vi "通过引用调用VI.vi"() -> ()   [LabVIEW 2013]
uses:
  <vilib>/Platform/TimedLoop/XDataNode/timing_clust.ctl
  <vilib>/Platform/TimedLoop/XDataNode/nitl_modes.ctl
  <vilib>/Platform/TimedLoop/XDataNode/wakeup.ctl
  <vilib>/Platform/TimedLoop/XDataNode/XDataNode.xnode
  <vilib>/Platform/TimedLoop/XDataNode/XDNodeRunTimeDep.lvlib
panel:
  in  "关闭引用":bool
  out "应用程序:所有内存中的VI":string[](array[string])
  out "result":dbl
  in  "y":dbl
  in  "x":dbl
  in  "停止":bool
  in  "VI":i32(listbox)
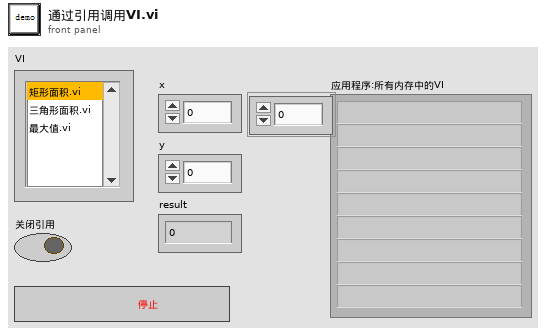
[diagram p1: front panel]
types:
  T1 = typedef "XDNodeRunTimeDep.lvlib/timing_clust.ctl" = cluster{"Expected End [f-1]":u64, "Actual End [f-1]":u64, "Finished Late? [f-1]":bool, "Expected End [i-1]":u64, "Actual End [i-1]":u64, "Finished Late? [i-1]":bool, "Expected Start [i]":u64, "Actual Start [i]":u64, "Expected Start [f]":u64, "Actual Start [f]":u64, "Source Name":string, "Structure Name":string, "Period":i64, "Deadline":i64, "Offset":i64, "Start":i64, "Priority":i32, "Timeout":i32, "Mode":T2, "Wakeup Reason":T3, "Error":errorcluster, "Source Type":string, "Secondary Source Type":string, "Global End Time":u64, "Global Start Time":u64, "Frame Duration":u64, "Iteration Duration":u64, "Assigned CPU":i32, "I/O Scan Engine Mode":u32}
  T2 = typedef "XDNodeRunTimeDep.lvlib/nitl_modes.ctl" = enum32{"No Change", "Process missed periods, maintain original phase", "Discard missed periods, maintain original phase", "Process missed periods, ignore original phase", "Discard missed periods, ignore original phase"}
  T3 = typedef "XDNodeRunTimeDep.lvlib/wakeup.ctl" = enum32{"Normal", "Aborted", "Asynchronous wakeup", "Timing source error", "Timed loop error", "Timeout"}
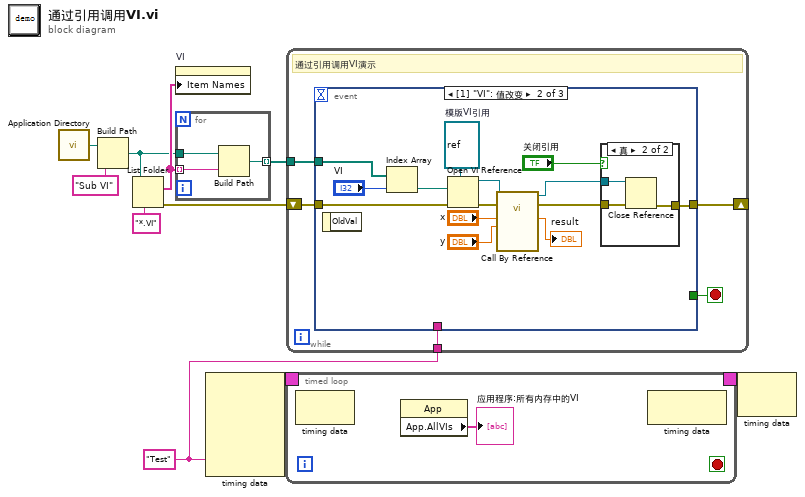
[diagram p0: block diagram]
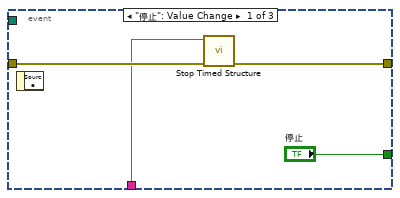
[diagram p2: hidden frame]
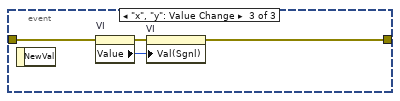
[diagram p4: hidden frame]
diagram:
  w1 = "Test" ("结构名称")
  n1 = call <vilib>:"Application Directory.vi"() -> ("Application Directory"=w10:path)
  n2 = Build Path(base path=w10, name or relative path="Sub VI" ("名称或相对路径")) -> (appended path=w6:path)
  n3 = List Folder(path=w6, pattern="*.VI" ("模式")) -> (filenames=w7:string[], error out=w4:errorcluster)  [unwired: 2 in, 2 out]
  n4 = property on="VI" class="LstBox (严格)"("Item Names"=w7) -> ()  [unwired: 2 in, 2 out]
  n5 = for {
    tunnel: w7 -> [w12] mode=indexing
    tunnel: w6 -> [w13]
    tunnel: [w11] -> w5 mode=indexing
    n6 = Build Path(base path=w13, name or relative path=w12) -> (appended path=w11:path)
  }
  n7 = node-c288(w1) -> (w3:T1)  [unwired: 4 in]
  n8 = timed-loop {
    timing: w3 -> [_]
    timing-out: [_] -> w2
    stop <- _ stop-if-true
    n9 = node-c288() -> ()  [unwired: 1 in, 1 out]
    n10 = property class="App"() -> ("App.AllVIs"=→"应用程序:所有内存中的VI":string[])  [unwired: 2 in, 2 out]
    n11 = node-c288() -> ()  [unwired: 1 in, 1 out]
  }
  n12 = while {
    shift-right: [w18] -> _
    shift-left: w4 -> [w19]
    tunnel: w5 -> [w20]
    tunnel: w1 -> [w17]
    stop <- w21 stop-if-true
    # "通过引用调用VI演示"
    n13 = event shown="[1] \"VI\": 值改变" {
      selector: _ -> [_ _ _]
      dyn-events: _ -> [_ _ _]
      timeout: _ -> [_ _ _]
      tunnel: ["停止" _ _] -> w21
      tunnel: w20 -> [_ w39 _]
      tunnel: w19 -> [w24 w30 w45]
      tunnel: [w23 w28 w44] -> w18
      tunnel: w17 -> [w22 _ _]
      event "停止": Value Change {
        n14 = event-data() -> ()  [unwired: 1 in, 1 out]
        n15 = call <vilib>:"Stop Timed Structure.vi"("error in (no error)"=w24, "name"=w22) -> ("error out"=w23:errorcluster)  [unwired: 9 in]
      }
      event "VI": Value Change {
        w33 = refnum<vi> refnum  # 模版VI引用
        n16 = event-data() -> ()  [unwired: 1 in, 1 out]
        n17 = Index Array(array=w39, index="VI") -> (element=w31:path)
        n18 = Open VI Reference(type specifier VI Refnum (for type only)=w33, vi path=w31, error in (no error)=w30) -> (vi reference=w32:refnum<vi>, error out=w37:errorcluster)  [unwired: 3 in]
        n19 = call-by-ref "?"(reference=w32, error in=w37, "y"="y", "x"="x") -> (reference out=w26:refnum<vi>, error out=w29:errorcluster, "result"=→"result":dbl)  [unwired: 9 in]
        n20 = case shown="真" "关闭引用" {
          tunnel: w29 -> [w40 w43]
          tunnel: [w40 w42] -> w28
          tunnel: w26 -> [_ w41]
          frame False {
          }
          frame True {
            n21 = Close Reference(reference=w41, error in (no error)=w43) -> (error out=w42:errorcluster)
          }
        }
      }
      event "x", "y": Value Change {
        n22 = event-data() -> ()  [unwired: 1 in, 1 out]
        n23 = property on="VI" class="LstBox (严格)"(error in=w45) -> (error out=w47:errorcluster, "Value"=w46:i32)  [unwired: 1 in, 1 out]
        n24 = property on="VI" class="LstBox (严格)"(error in=w47, "Val(Sgnl)"=w46) -> (error out=w44:errorcluster)  [unwired: 1 in, 1 out]
      }
    }
  }
  n25 = node-c288(w2) -> ()  [unwired: 1 out]
